vi "Save MC data.vi"(6 "Stop":bool, 7 "Initialise":bool, 8 "error in (no error)":errorcluster, 11 "Input":dbl[](array[numeric])) -> (0 "error out":errorcluster, 3 "MC Data Save ON":bool)   [LabVIEW 2020]
uses:
  Typedefs/Read Write Enum.ctl
panel:
  out "Test GraphData Path":path
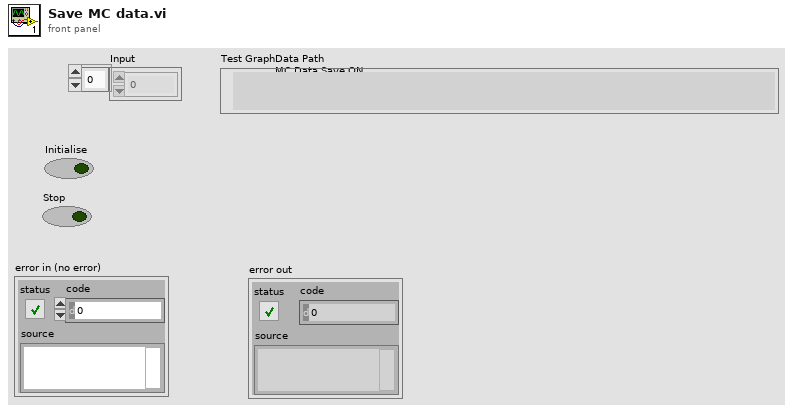
[diagram p1: front panel]
types:
  T1 = typedef "Read Write Enum.ctl" = enum16{"Read", "Write"}
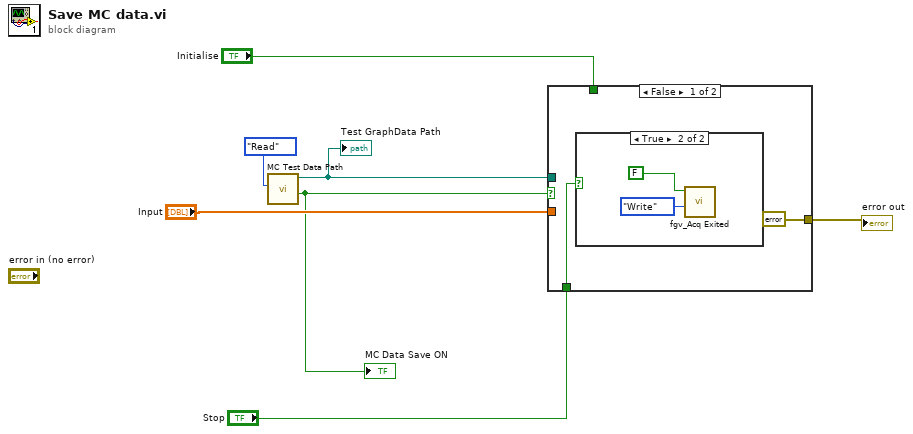
[diagram p0: block diagram]
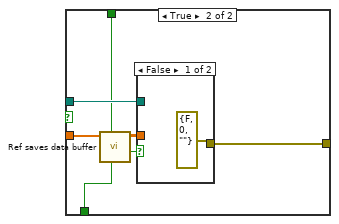
[diagram p3: hidden frame]
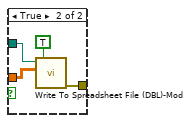
[diagram p4: hidden frame]
diagram:
  n1 = call "MC Test Data Path.vi"("State"=enum16{"Initialise", "Write", "Read"}."Read") -> ("Save Test Data"=w2:bool, "Test GraphData Path"=w1:path)  [unwired: 8 in, 1 out]
  "MC Data Save ON" <- w2
  "Test GraphData Path" <- w1
  n2 = case shown="False" w2 {
    tunnel: w1 -> [_ w18]
    tunnel: [errorcluster {"status"=FALSE, "code"=0, "source"=""} ("error out") w17] -> w6
    tunnel: "Input" -> [_ w16]
    tunnel: "Initialise" -> [_ w14]
    tunnel: "Stop" -> [w8 w13]
    frame False {
      n3 = case shown="True" w8 {
        frame False {
        }
        frame True {
          n4 = call "fgv_Acq Exited.vi"("Function"=Read_Write_Enum."Write", "Acquisition completed"=FALSE) -> ()  [unwired: 8 in, 2 out]
        }
      }
    }
    frame True {
      n5 = call "Ref saves data buffer.vi"("Stop"=w13, "Initialise"=w14, "Array in"=w16) -> ("Save data"=w12:bool, "Array out"=w15:dbl[][])  [unwired: 7 in]
      n6 = case shown="False" w12 {
        tunnel: w18 -> [_ w23]
        tunnel: [errorcluster {"status"=FALSE, "code"=0, "source"=""} ("error out") w21] -> w17
        tunnel: w15 -> [_ w20]
        frame False {
        }
        frame True {
          n7 = call <userlib>:"Write To Spreadsheet File (DBL)-Mod.vi"("append to file? (new file:F)"=TRUE, "2D data"=w20, "file path (dialog if empty)"=w23) -> ("error out"=w21:errorcluster)  [unwired: 7 in, 1 out]
        }
      }
    }
  }
  "error out" <- w6
